vi "Remove Key.vi"(7 "Section":string, 8 "error in (no error)":errorcluster, 10 "Key":string, 11 "Ini Path in":path) -> (0 "error out":errorcluster, 1 "Key Found?":bool, 3 "Ini Path out":path)   [LabVIEW 2018, in "Cfg.lvlib"]
uses:
  Cfg.lvlib
  Action.ctl
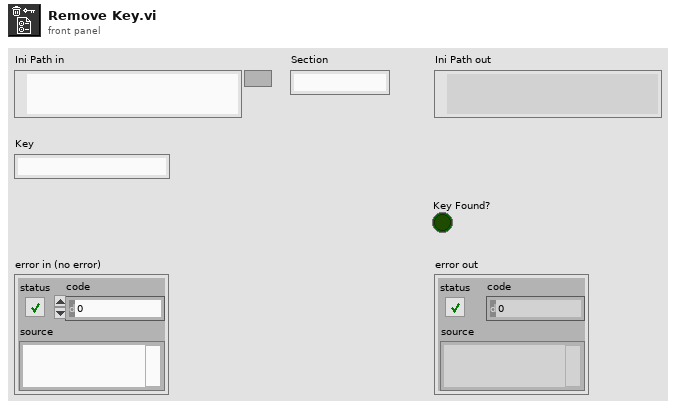
[diagram p1: front panel]
types:
  T1 = typedef "Cfg.lvlib/Action.ctl" = enum8{"noop", "new", "read_or_create", "read", "write", "remove", "keys", "sections", "remove_section", "import", "export", "get", "set", "pop", "add", "list", "list_sections", "pop_section"}
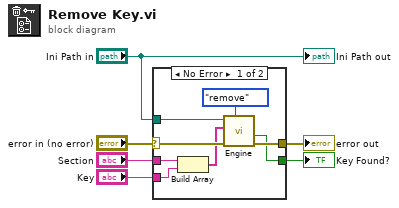
[diagram p0: block diagram]
diagram:
  n1 = case shown="No Error" "error in (no error)" {
    selector: "error in (no error)" -> [w14 w15]
    tunnel: "Ini Path in" -> [w12 _]
    tunnel: [w11 w15] -> w4
    tunnel: "Section" -> [w10 _]
    tunnel: [w8 _] -> w2
    tunnel: "Key" -> [w7 _]
    frame No Error {
      n2 = Build Array(w10, w7) -> (w9:string[])
      n3 = call "Engine.vi"("Action"=Action."remove", "error in (no error)"=w14, "skvc in"=w9, "INI Path in"=w12) -> ("error out"=w11:errorcluster, "Found?"=w8:bool)  [unwired: 4 in, 2 out]
    }
    frame Error {
    }
  }
  "error out" <- w4
  "Key Found?" <- w2
  "Ini Path out" <- "Ini Path in"
